vi "DispalyStatus.vi"(0 "Status In":bool, 1 "Caption Array":string[](array[string])=["CONTROLLER\nCONNECTED", "CONTROLLER\nDISCONNECTED"], 2 "Time Index":i32, 3 "error in":errorcluster, 4 "Boolean Status Ref":refnum<vi>) -> (7 "Status Displayed":bool, 10 "error out":errorcluster)   [LabVIEW 2016]
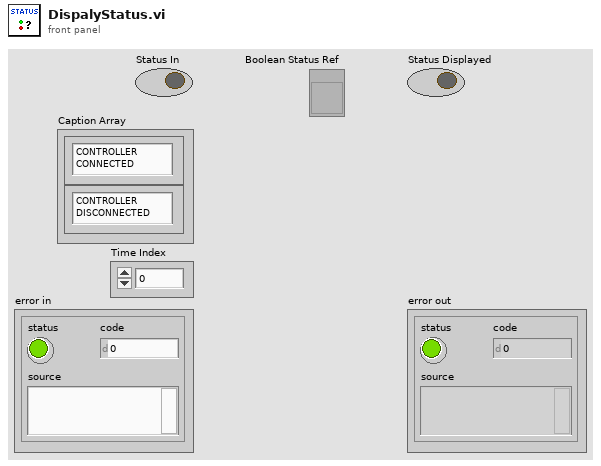
[diagram p1: front panel]
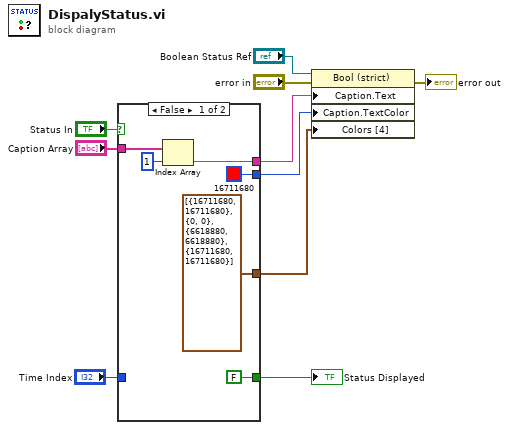
[diagram p0: block diagram]
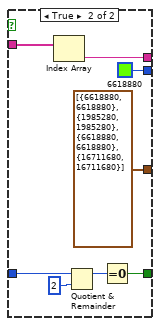
[diagram p2: hidden frame]
diagram:
  n1 = case shown="False" "Status In" {
    tunnel: [FALSE w22] -> w4
    tunnel: [u32 16711680 ("Color Box") u32 6618880 ("Color Box")] -> w6
    tunnel: [w12 w17] -> w7
    tunnel: [cluster{"Color Box":u32, "Color Box 2":u32}[] [{"Color Box"=16711680, "Color Box 2"=16711680}, {"Color Box"=0, "Color Box 2"=0}, {"Color Box"=6618880, "Color Box 2"=6618880}, {"Color Box"=16711680, "Color Box 2"=16711680}] ("Colors [4]") cluster{"Color Box":u32, "Color Box 2":u32}[] [{"Color Box"=6618880, "Color Box 2"=6618880}, {"Color Box"=1985280, "Color Box 2"=1985280}, {"Color Box"=6618880, "Color Box 2"=6618880}, {"Color Box"=16711680, "Color Box 2"=16711680}] ("Colors [4]")] -> w8
    tunnel: "Time Index" -> [_ w19]
    tunnel: "Caption Array" -> [w13 w18]
    frame False {
      n2 = Index Array(array=w13, index=1) -> (element=w12:string)
    }
    frame True {
      n3 = Index Array(array=w18) -> (element=w17:string)  [unwired: 1 in]
      n4 = Quotient & Remainder(x=w19, y=2) -> (x-y*floor(x/y)=w23:i32)  [unwired: 1 out]
      n5 = Equal To 0?(x=w23) -> (x = 0?=w22:bool)
    }
  }
  "Status Displayed" <- w4
  n6 = property class="Bool (strict)"(reference="Boolean Status Ref", error in="error in", "Caption.Text"=w7, "Caption.TextColor"=w6, "Colors [4]"=w8) -> (error out=→"error out":errorcluster)  [unwired: 1 out]
